vi "Connect Multi Frame_SPI.vi"(7 "SPI_Mode":T1, 8 "error in (no error)":errorcluster, 10 "Timeset between frms":u32=50, 11 "SPI Frame Array":refnum<class "SPI_Frame_Root.lvclass">[](array[class])) -> (0 "error out":errorcluster, 3 "Connected Frame Contents":string)   [LabVIEW 2018, in "DigiPattern_Generator.lvclass"]
uses:
  DigiPattern_Generator.lvclass
  SPI/SPI Frame Root/SPI_Frame_Root.lvclass
  SPI/Config Read SPI/SPI_Mode.ctl
  SPI/SPI Frame Root/SPI_Frame_Root.lvclass/SPI_Frame_Root.ctl
  BML_Frame_Root/Special Frame.ctl
  BML_Frame_Root/BML_Frame_Root.lvclass
  SPI/Config Read SPI/Config_Read_SPI.lvclass
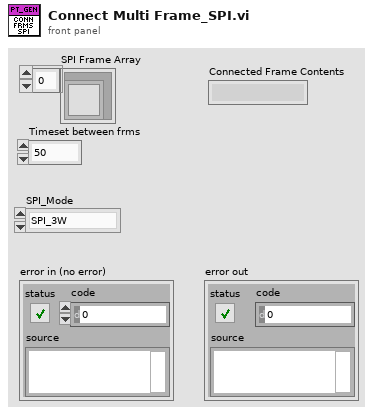
[diagram p1: front panel]
types:
  T1 = typedef "Config_Read_SPI.lvclass/SPI_Mode.ctl" = enum16{"SPI_3W", "SPI_4W"}
  T2 = typedef "BML_Frame_Root.lvclass/Special Frame.ctl" = enum16{"Sync Header", "Protocol Header", "SW Trig", "SetID State", "Out SetID State", "SW Reset", "Wait", "SPI 4W FRM Start", "SPI 4W Wait", "SPI 4W FRM End", "SPI 4W Write Cmd", "SPI RD Collect Cmd", "SPI RD Value Cmd", "SPI 3W FRM Start", "SPI 3W Write Cmd", "SPI 3W FRM End", "SPI 3W Wait", "SPI 3W RD Cmd"}
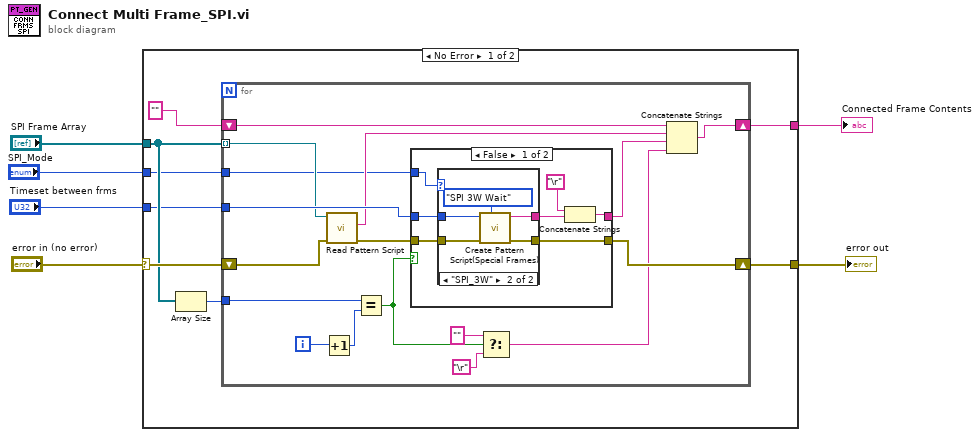
[diagram p0: block diagram]
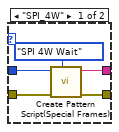
[diagram p2: hidden frame]
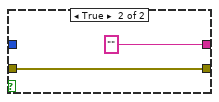
[diagram p3: hidden frame]
diagram:
  n1 = case shown="No Error" "error in (no error)" {
    selector: "error in (no error)" -> [w12 w51]
    tunnel: "SPI Frame Array" -> [w11 _]
    tunnel: [w13 w51] -> w5
    tunnel: [w9 _] -> w3
    tunnel: "Timeset between frms" -> [w8 _]
    tunnel: "SPI_Mode" -> [w7 _]
    frame No Error {
      n2 = Array Size(array=w11) -> (size(s)=w10:i32)
      n3 = for {
        tunnel: w11 -> [w19] mode=indexing
        shift-right: [w24] -> w13
        shift-left: w12 -> [w17]
        shift-right: [w31] -> w9
        shift-left: "" -> [w30]
        tunnel: w10 -> [w23]
        tunnel: w8 -> [w20]
        tunnel: w7 -> [w15]
        i -> [w29]
        n4 = Increment(x=w29) -> (x+1=w28:i32)
        n5 = call "Read Pattern Script.vi"("error in (no error)"=w17, "SPI_Frame_Root in"=w19) -> ("error out"=w16:errorcluster, "Pattern Script"=w18:string)  [unwired: 7 in, 1 out]
        n6 = Equal?(x=w23, y=w28) -> (x = y?=w25:bool)
        n7 = case shown="False" w25 {
          tunnel: w16 -> [w38 w49]
          tunnel: [w37 w49] -> w24
          tunnel: w20 -> [w36 _]
          tunnel: [w34 "" ("string out")] -> w21
          tunnel: w15 -> [w32 _]
          frame False {
            n8 = case shown="\"SPI_3W\"" w32 {
              tunnel: w38 -> [w43 w48]
              tunnel: [w42 w47] -> w37
              tunnel: w36 -> [w41 w46]
              tunnel: [w40 w45] -> w35
              frame "SPI_4W" {
                n9 = call "Create Pattern Script(Special Frames).vi"("Special Frame Type"=Special_Frame."SPI 4W Wait", "error in (no error)"=w43, "Num of Timeset"=w41) -> ("error out"=w42:errorcluster, "string out"=w40:string)  [unwired: 7 in]
              }
              frame "SPI_3W" {
                n10 = call "Create Pattern Script(Special Frames).vi"("Special Frame Type"=Special_Frame."SPI 3W Wait", "error in (no error)"=w48, "Num of Timeset"=w46) -> ("error out"=w47:errorcluster, "string out"=w45:string)  [unwired: 7 in]
              }
            }
            n11 = Concatenate Strings("\r", w35) -> (w34:string)
          }
          frame True {
          }
        }
        n12 = Select(t="", s=w25, f="\r") -> (s? t:f=w22:string)
        n13 = Concatenate Strings(w30, w18, w21, w22) -> (w31:string)
      }
    }
    frame Error {
    }
  }
  "error out" <- w5
  "Connected Frame Contents" <- w3
